vi "WPI_CANJaguar_Enable.vi"(8 "error in (no error)":errorcluster, 10 "Encoder Initial Position":dbl, 11 "CAN MotorDevRef":T1={"DeviceStatus"={"status"=FALSE, "code"=0, "source"=""}, "Type"=enum."PWM", "PWM"={"PWM Channel"=enum."Invalid", "DeadBand"={"Name"="", "maxPositivePwm"=0, "minPositivePwm"=0, "centerPwm"=0, "maxNegativePwm"=0, "minNegativePwm"=0, "angularRange"=0}}, "CAN"={"Device Number"=0, "SetOutput VI Ref"=variant(enum8{"Percent VBus", "Current", "Speed", "Position", "Voltage"} enum."Percent VBus"), "GetOutput VI Ref"=variant(refnum<k1> refnum), "Enable VI Ref"=variant(dbl 12.0), "Disable VI Ref"=variant(enum8{"Percent VBus", "Speed", "Position", "Slave", "Unchanged / Invalid", "Voltage Compensation", "Current", "Motion Profile"} enum."Percent VBus"), "Data"=variant}, "Invert"=FALSE}) -> (0 "error out":errorcluster, 3 "CAN MotorDevRef":T1={"DeviceStatus"={"status"=FALSE, "code"=0, "source"=""}, "Type"=enum."PWM", "PWM"={"PWM Channel"=enum."Invalid", "DeadBand"={"Name"="", "maxPositivePwm"=0, "minPositivePwm"=0, "centerPwm"=0, "maxNegativePwm"=0, "minNegativePwm"=0, "angularRange"=0}}, "CAN"={"Device Number"=0, "SetOutput VI Ref"=variant(enum8{"Percent VBus", "Current", "Speed", "Position", "Voltage"} enum."Percent VBus"), "GetOutput VI Ref"=variant(refnum<k1> refnum), "Enable VI Ref"=variant(dbl 12.0), "Disable VI Ref"=variant(enum8{"Percent VBus", "Speed", "Position", "Slave", "Unchanged / Invalid", "Voltage Compensation", "Current", "Motion Profile"} enum."Percent VBus"), "Data"=variant}, "Invert"=FALSE})   [LabVIEW 2016]
doc: "Enable the closed loop controller in the <B>Control Mode</B> that was specified in <B>Open</B> on a CAN Jaguar. You must also call this VI after calling the <B>Change Mode</B> VI to start the closed loop controller.\n\nThis software is licensed. Open the labview\\readme\\WPI Robotics Library Open Source License.txt file for more information."
uses:
  <vilib>/Rock Robotics/WPI/MotorControl/WPI_MotorControlDeviceRef.ctl
  <vilib>/Rock Robotics/WPI/MotorControl/WPI_MotorControlType.ctl
  <vilib>/Rock Robotics/SystemInterfaces/DIO/FPGA_DIOPWMChannel.ctl
  <vilib>/Rock Robotics/WPI/PWM/WPI_PWMDeadband.ctl
  <vilib>/Rock Robotics/WPI/ThirdParty/CanMotor/CAN Jaguar/SubVIs/WPI_CANJaguar_RefNumData.ctl
  <vilib>/Rock Robotics/WPI/ThirdParty/CanMotor/CAN Jaguar/SubVIs/WPI_CANJaguar_ControlMode.ctl
  <vilib>/Rock Robotics/WPI/ThirdParty/CanMotor/CAN Jaguar/SubVIs/WPI_CAN_TokenMessageIDs.ctl
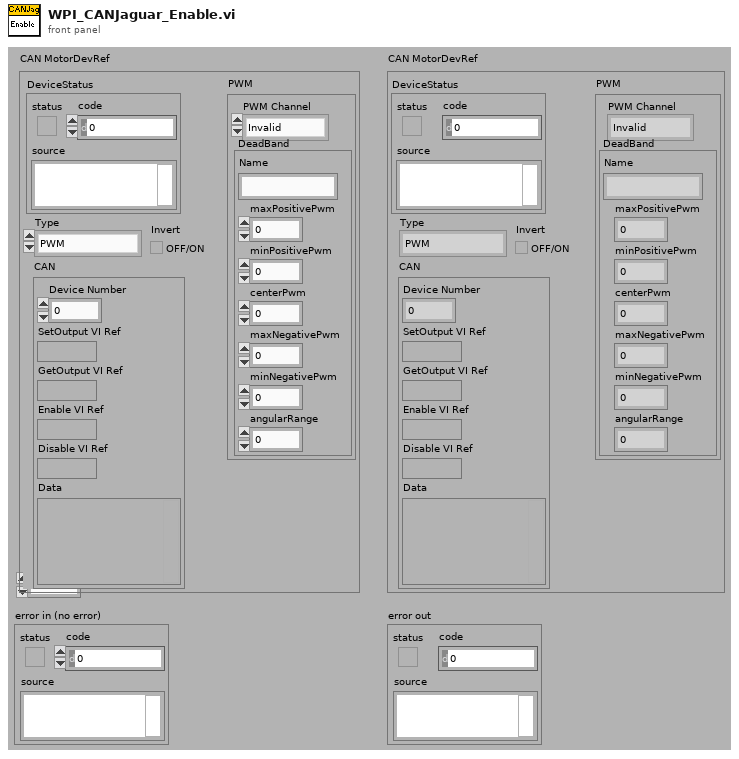
[diagram p1: front panel]
types:
  T1 = typedef "WPI_MotorControlDeviceRef.ctl" = cluster{"DeviceStatus":errorcluster, "Type":T2, "PWM":cluster{"PWM Channel":T3, "DeadBand":T4}, "CAN":cluster{"Device Number":u8, "SetOutput VI Ref":variant, "GetOutput VI Ref":variant, "Enable VI Ref":variant, "Disable VI Ref":variant, "Data":variant}, "Invert":bool}
  T2 = typedef "WPI_MotorControlType.ctl" = enum16{"PWM", "CAN"}
  T3 = typedef "FPGA_DIOPWMChannel.ctl" = enum8{"PWM 0", "PWM 1", "PWM 2", "PWM 3", "PWM 4", "PWM 5", "PWM 6", "PWM 7", "PWM 8", "PWM 9", "PWM MXP 0", "PWM MXP 1", "PWM MXP 2", "PWM MXP 3", "PWM MXP 4", "PWM MXP 5", "PWM MXP 6", "PWM MXP 7", "PWM MXP 8", "PWM MXP 9", "Invalid"}
  T4 = typedef "WPI_PWMDeadband.ctl" = cluster{"Name":string, "maxPositivePwm":i32, "minPositivePwm":i32, "centerPwm":i32, "maxNegativePwm":i32, "minNegativePwm":i32, "angularRange":u16}
  T5 = enum16{"big-endian, network order", "native, host order", "little-endian"}
  T6 = typedef "WPI_CANJaguar_RefNumData.ctl" = cluster{"CAN.Max Vout":dbl, "Control Mode":T7, "semaphore":T8}
  T7 = typedef "WPI_CANJaguar_ControlMode.ctl" = enum8{"Percent VBus", "Current", "Speed", "Position", "Voltage"}
  T8 = typedef "Semaphore RefNum" = refnum<k1>
  T9 = typedef "WPI_CAN_TokenMessageIDs.ctl" = u32
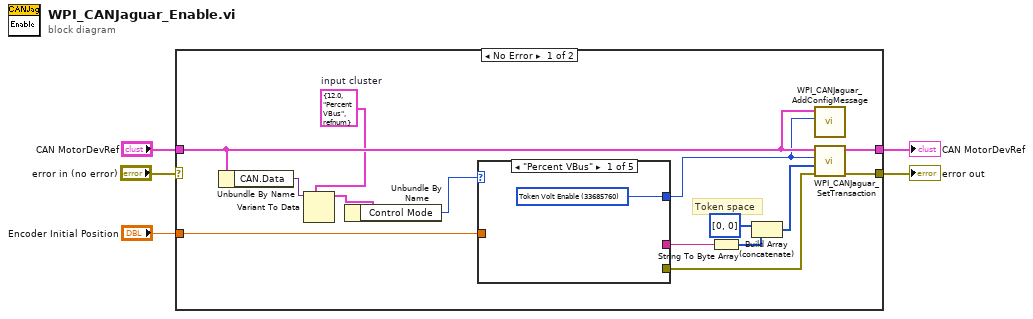
[diagram p0: block diagram]
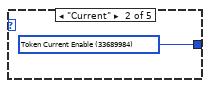
[diagram p2: hidden frame]
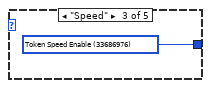
[diagram p3: hidden frame]
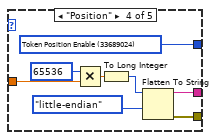
[diagram p4: hidden frame]
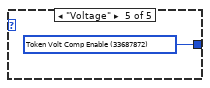
[diagram p5: hidden frame]
diagram:
  n1 = case shown="No Error" "error in (no error)" {
    selector: "error in (no error)" -> [_ w33]
    tunnel: "CAN MotorDevRef" -> [w18 w32]
    tunnel: [w16 w32] -> w4
    tunnel: [w17 w33] -> w3
    tunnel: "Encoder Initial Position" -> [w19 _]
    frame No Error {
      w8 = T6 {"CAN.Max Vout"=12.0, "Control Mode"=enum."Percent VBus", "semaphore"=refnum}  # input cluster
      # "Token space"
      n2 = Unbundle By Name(w18) -> ("CAN.Data"=w9:variant)
      n3 = Variant To Data(type=w8, Variant=w9) -> (data=w7:T6)  [unwired: 1 in, 1 out]
      n4 = Unbundle By Name(w7) -> ("Control Mode"=w6:T7)
      n5 = case shown="\"Percent VBus\"" w6 {
        tunnel: [w20 w21 w22 w30 w31] -> w10
        tunnel: w19 -> [_ _ _ w29 _]
        tunnel: [_ _ _ w26 _] -> w12
        tunnel: [_ _ _ w23 _] -> w14
        frame "Percent VBus" {
          w20 = T9 33685760 items=["Token Volt Enable"=33685760, "Token Volt Set"=33685824, "Token Volt Set No Ack"=33685952, "Token Speed Enable"=33686976, "Token Speed Set"=33687040, "Token Speed Set No Ack"=33687168, "Token Volt Comp Enable"=33687872, "Token Volt Comp Set"=33687936, "Token Volt Comp Set No Ack"=33688064, "Token Position Enable"=33689024, "Token Position Set"=33689088, "Token Position Set No Ack"=33689216, "Token Current Enable"=33689984, "Token Current Set"=33690048, "Token Current Set No Ack"=33690176] ("CAN Token Message IDs")
        }
        frame "Current" {
          w21 = T9 33689984 items=["Token Volt Enable"=33685760, "Token Volt Set"=33685824, "Token Volt Set No Ack"=33685952, "Token Speed Enable"=33686976, "Token Speed Set"=33687040, "Token Speed Set No Ack"=33687168, "Token Volt Comp Enable"=33687872, "Token Volt Comp Set"=33687936, "Token Volt Comp Set No Ack"=33688064, "Token Position Enable"=33689024, "Token Position Set"=33689088, "Token Position Set No Ack"=33689216, "Token Current Enable"=33689984, "Token Current Set"=33690048, "Token Current Set No Ack"=33690176] ("CAN Token Message IDs")
        }
        frame "Speed" {
          w22 = T9 33686976 items=["Token Volt Enable"=33685760, "Token Volt Set"=33685824, "Token Volt Set No Ack"=33685952, "Token Speed Enable"=33686976, "Token Speed Set"=33687040, "Token Speed Set No Ack"=33687168, "Token Volt Comp Enable"=33687872, "Token Volt Comp Set"=33687936, "Token Volt Comp Set No Ack"=33688064, "Token Position Enable"=33689024, "Token Position Set"=33689088, "Token Position Set No Ack"=33689216, "Token Current Enable"=33689984, "Token Current Set"=33690048, "Token Current Set No Ack"=33690176] ("CAN Token Message IDs")
        }
        frame "Position" {
          w30 = T9 33689024 items=["Token Volt Enable"=33685760, "Token Volt Set"=33685824, "Token Volt Set No Ack"=33685952, "Token Speed Enable"=33686976, "Token Speed Set"=33687040, "Token Speed Set No Ack"=33687168, "Token Volt Comp Enable"=33687872, "Token Volt Comp Set"=33687936, "Token Volt Comp Set No Ack"=33688064, "Token Position Enable"=33689024, "Token Position Set"=33689088, "Token Position Set No Ack"=33689216, "Token Current Enable"=33689984, "Token Current Set"=33690048, "Token Current Set No Ack"=33690176] ("CAN Token Message IDs")
          n6 = Multiply(x=u32 65536, y=w29) -> (x*y=w27:dbl)
          n7 = To Long Integer(number=w27) -> (32bit integer=w24:i32)
          n8 = Flatten To String(anything=w24, byte order (0:big-endian, network order)=T5."little-endian") -> (data string=w23:string, error out=w26:errorcluster)  [unwired: 2 in, 1 out]
        }
        frame "Voltage" {
          w31 = T9 33687872 items=["Token Volt Enable"=33685760, "Token Volt Set"=33685824, "Token Volt Set No Ack"=33685952, "Token Speed Enable"=33686976, "Token Speed Set"=33687040, "Token Speed Set No Ack"=33687168, "Token Volt Comp Enable"=33687872, "Token Volt Comp Set"=33687936, "Token Volt Comp Set No Ack"=33688064, "Token Position Enable"=33689024, "Token Position Set"=33689088, "Token Position Set No Ack"=33689216, "Token Current Enable"=33689984, "Token Current Set"=33690048, "Token Current Set No Ack"=33690176] ("CAN Token Message IDs")
        }
      }
      n9 = String To Byte Array(string=w14) -> (unsigned byte array=w13:u8[])
      n10 = Build Array (concatenate)(u8[] [0, 0] ("data"), w13) -> (w11:u8[])
      n11 = call <vilib>:"WPI_CANJaguar_AddConfigMessage.vi"("Message ID"=w10, "CAN Jaguar Ref"=w18) -> ()  [unwired: 10 in]
      n12 = call <vilib>:"WPI_CANJaguar_SetTransaction.vi"("error in"=w12, "Data"=w11, "Message ID"=w10, "CAN Jaguar Ref"=w18) -> ("error out"=w17:errorcluster, "CAN Jaguar Ref Out"=w16:T1)  [unwired: 6 out]
    }
    frame Error {
    }
  }
  "error out" <- w3
  "CAN MotorDevRef" <- w4
